vi "5_1.vi"() -> ()   [LabVIEW 2025, in "2023.lvlib"]
uses:
  2023.lvlib
  <vilib>/Utility/miscctls.llb/LVMapReplaceAction.ctl
  <userlib>/_OpenG.lib/string/string.llb/openg_string.lvlib
panel:
  out "Numeric 2":i32
  out "Map":T1(c390)
  out "64bit integer":i64[](array[numeric])
  out "Numeric":i32
  out "min value":i64
  out "subarray":i64[](array[numeric])
  out "Array 4":i64[][](array[numeric])
  out "Array":string[](array[string])
  out "lines":string[](array[string])
  in  "DEMO / REAL input":bool
  # "too low"
  # "485430760"
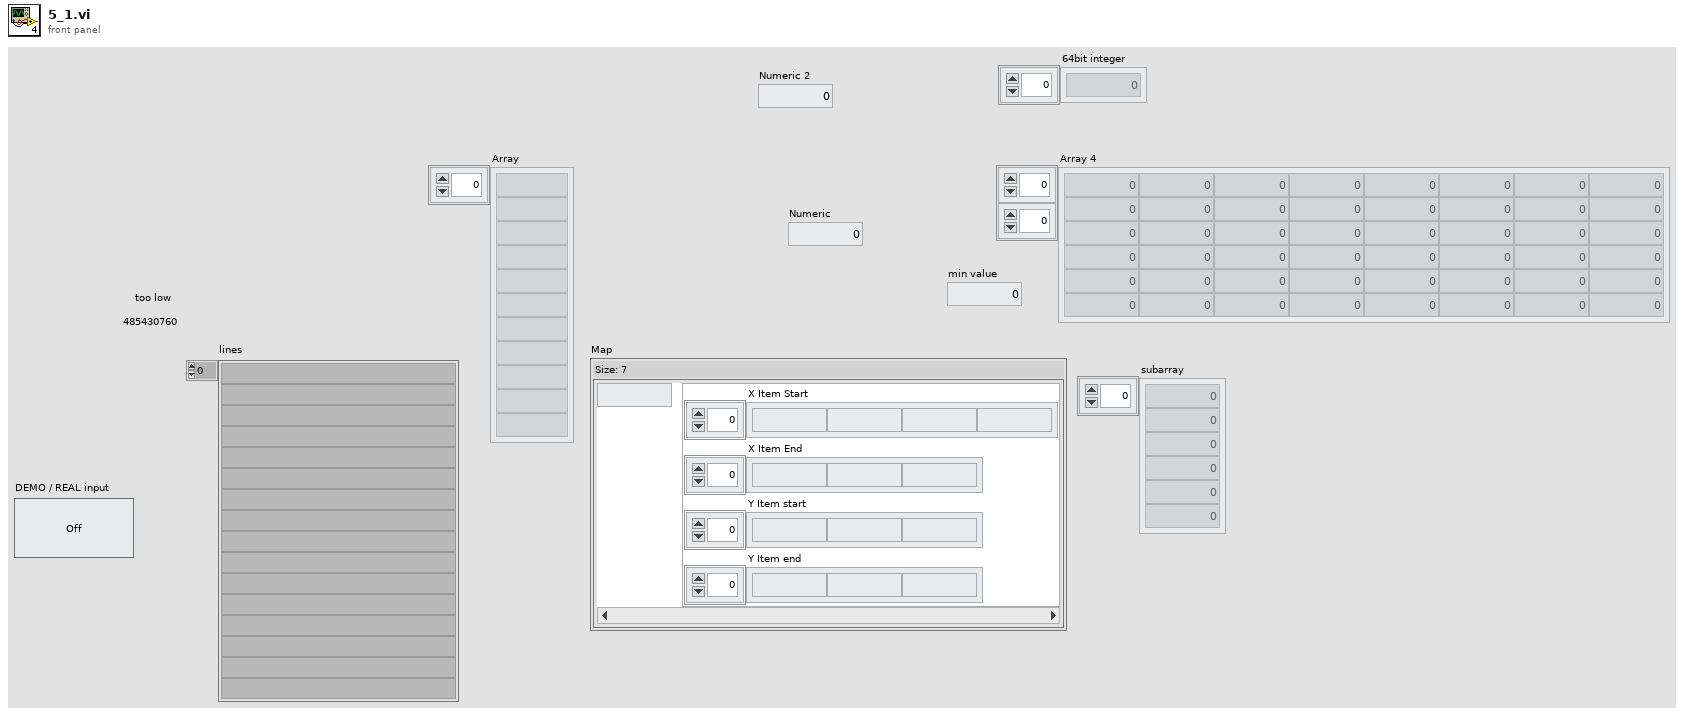
[diagram p1: front panel]
types:
  T1 = map{i32, cluster{"X Item Start":i64[], "X Item End":i64[], "Y Item start":i64[], "Y Item end":i64[]}}
  T2 = typedef "LVMapReplaceAction.ctl" = enum32{"Modify Entry only if found", "Add or Modify Entry", "Delete Entry"}
  T3 = cluster{"X Item Start":i64[], "X Item End":i64[], "Y Item start":i64[], "Y Item end":i64[]}
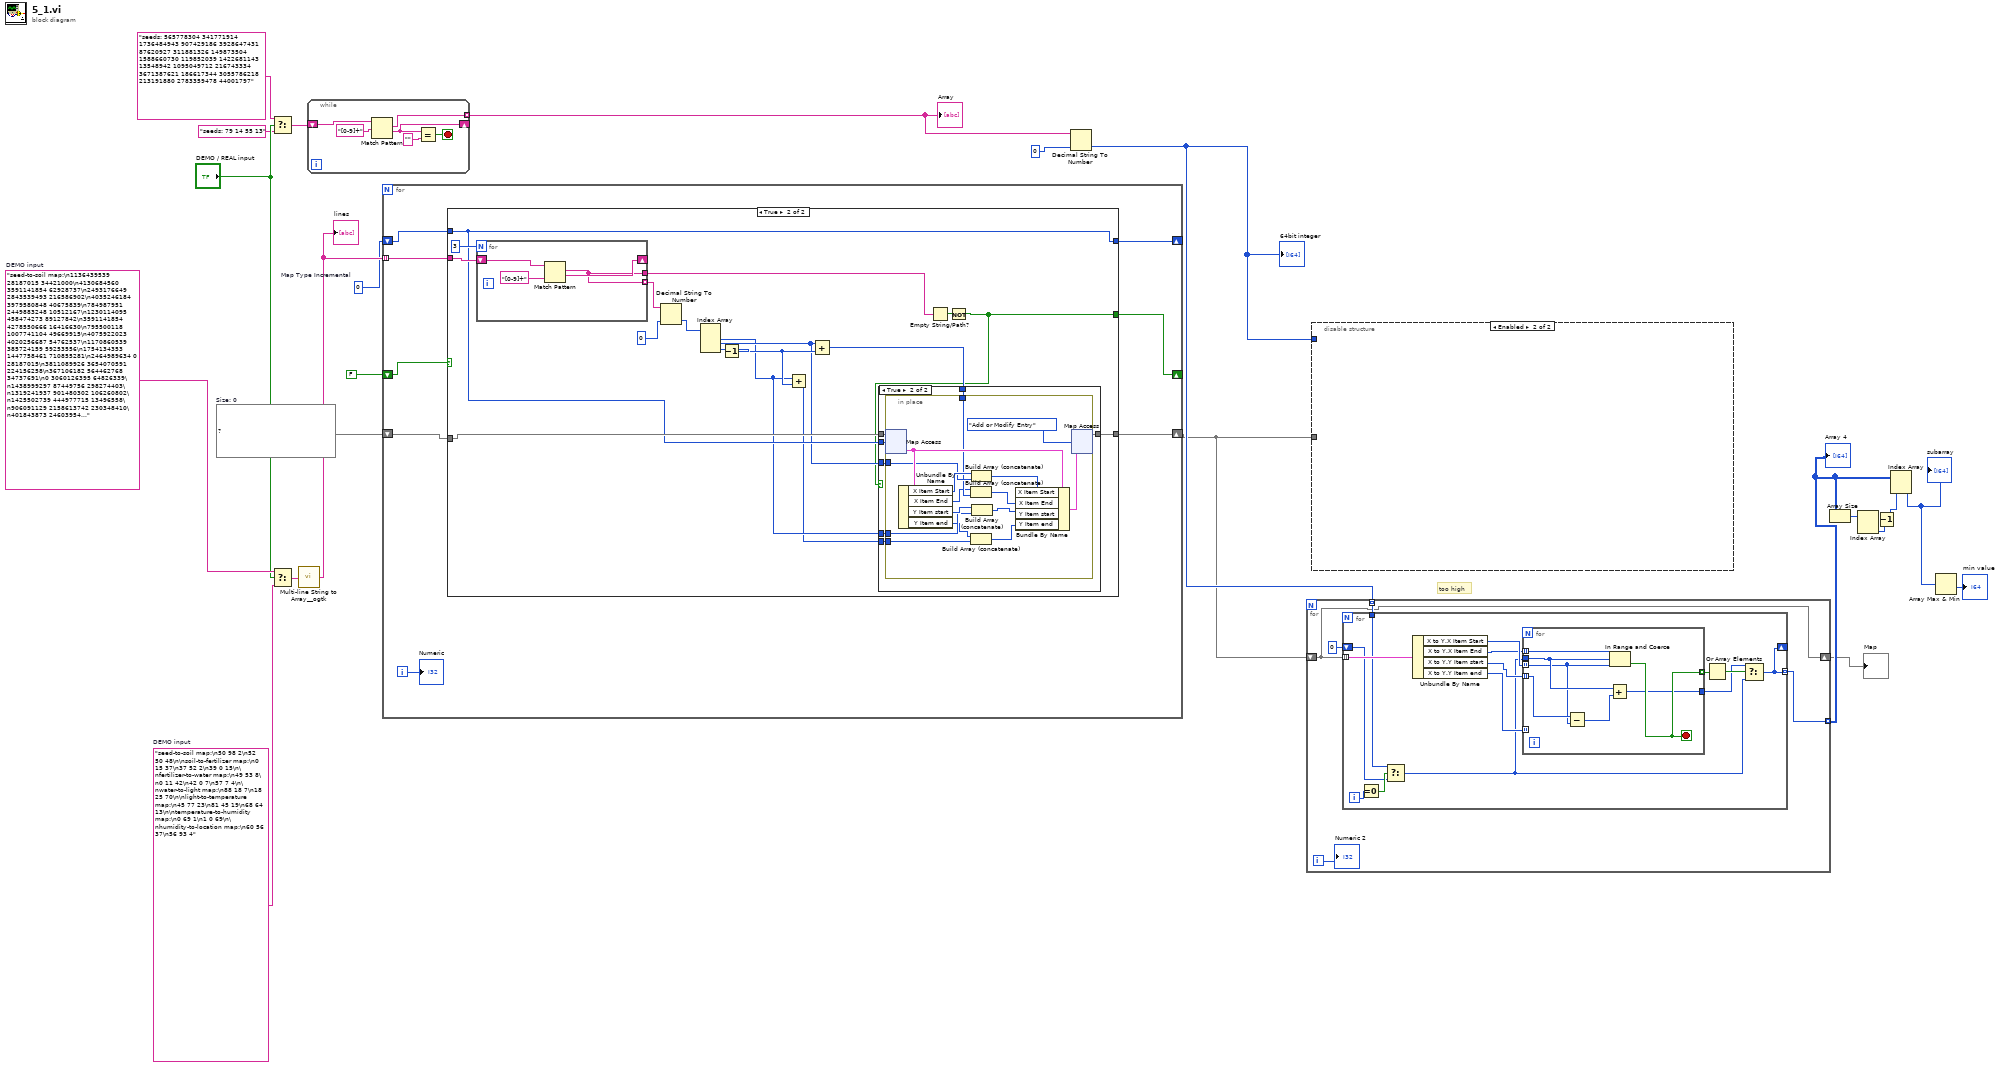
[diagram p0: block diagram]
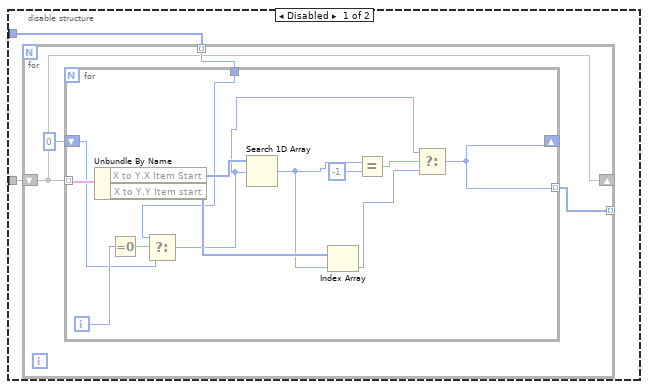
[diagram p2: hidden frame]
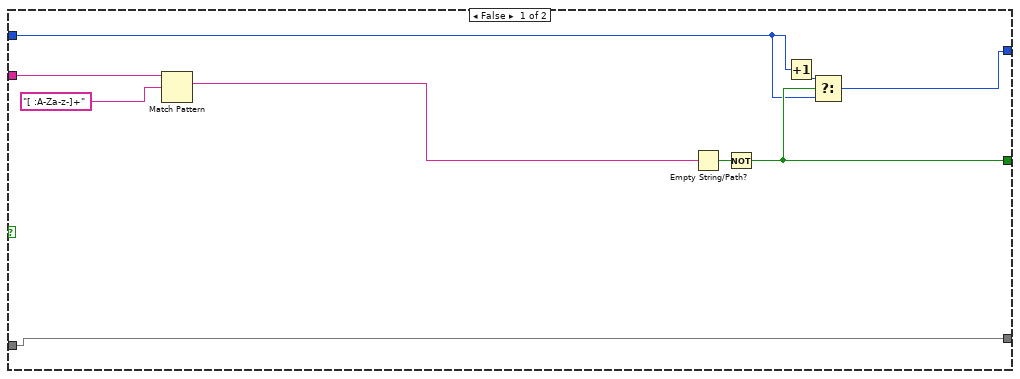
[diagram p3: hidden frame]
diagram:
  w11 = 0  # Map Type Incremental
  w13 = T1 {}  # Size: 0
  w22 = "seed-to-soil map:\n1136439539 28187015 34421000\n4130684560 3591141854 62928737\n2493176649 2843539493 216586902\n4035246184 3979580848 40675839\n784987951 2449883248 10512167\n1230114095 458474273 89127842\n3591141854 4278550666 16416630\n795500118 1007741104 49669915\n4075922023 4020256687 54762537\n1170860539 385724159 59253556\n1754134353 1447758461 710855281\n2464989634 0 28187015\n3811089926 3654070591 224156258\n367106182 564462768 34737691\n0 3060126395 64826339\n1438999297 87449756 298274403\n1319241937 901480302 106260802\n1425502739 444977715 13496558\n906091129 2158613742 230348410\n401843873 2460395415 383144078\n1737273700 547602115 16860653\n64826339 599200459 302279843\n2709763551 1057411019 390347442\n845170033 2388962152 60921096\n3607558484 4075019224 203531442\n3100110993 3124952734 265337006\n4193613297 3878226849 101353999\n3365447999 62608015 24841741\n\nsoil-to-fertilizer map:\n2997768542 2385088490 141138894\n2483957796 2361581050 23507440\n98641524 1346083581 385280737\n3138907436 2256873732 8670947\n0 2158232208 98641524\n3147578383 2265544679 96036371\n1035235183 2879344429 108036359\n2567031012 2526227384 63435416\n740156227 2589662800 180702628\n2630466428 1790930094 367302114\n1029837856 0 5397327\n1143271542 5397327 1340686254\n483922261 2987380788 256233966\n2507465236 1731364318 59565776\n920858855 2770365428 108979001\n\nfertilizer-to-water map:\n1539871014 1431400479 38399903\n4189242304 3947275099 105724992\n2012473116 0 61612686\n3673653298 3769966020 177309079\n25380533 833117788 21807501\n143369400 1411638591 19761888\n2698209531 61612686 40666379\n401367210 2888296065 27849039\n3850962377 4057978463 170640183\n1076364770 854925289 39443942\n0 2048878915 25380533\n2682826842 1483785677 15382689\n4026580932 4228618646 66348650\n790899137 2074259448 70405647\n2738875910 2609016218 230235412\n2090748148 1854132037 12185242\n163131288 1499168366 238235922\n1115808712 3002097202 63461270\n545943998 1215727887 195910704\n4092929582 3673653298 96312722\n1000530579 3065558472 75834191\n2074085802 2916145104 16662346\n429216249 1737404288 116727749\n1578270917 2174814019 434202199\n2969111322 102279065 44844471\n1179269982 669063687 164054101\n2463111278 507301424 161762263\n741854702 2839251630 49044435\n3013955793 894369231 236513741\n861304784 2144665095 30148924\n1525885719 1469800382 13985295\n132032949 2932807450 11336451\n2102933390 147123536 360177888\n47188034 1130882972 84844915\n4021602560 4053000091 4978372\n2624873541 2944143901 57953301\n891453708 3141392663 109076871\n1343324083 1866317279 182561636\n\nwater-to-light map:\n1509583382 1639808290 20361832\n3841220400 2799952377 116887408\n1472887638 3349716751 36695744\n1375316591 4197396249 97571047\n1030032900 38536653 44339012\n3776233310 1557050237 64987090\n1857053855 3386412495 71799907\n2963593546 2694182899 38493443\n3758462347 1622037327 17770963\n1018869652 82875665 11163248\n1308040556 2732676342 67276035\n1928853762 3953749938 243646311\n2488961036 3503789336 239267964\n3562290347 3458212402 6096433\n3568386780 1308040556 190075567\n2728229000 1997029610 235364546\n215668494 0 38536653\n1646361217 3743057300 109790942\n1529945214 3233300748 116416003\n1756152159 3852848242 100901696\n3958107808 1660170122 336859488\n3503356233 1498116123 58934114\n254205147 552157437 522214475\n3002086989 3464308835 39480501\n776419622 94038913 242450030\n2172500073 2916839785 316460963\n0 336488943 215668494\n3041567490 2232394156 461788743\n\nlight-to-temperature map:\n3498288578 2645051323 42074132\n608593503 673232568 65024140\n0 1287033796 108723708\n3979313387 3634135302 315653909\n2652759587 3018896130 103365881\n1093544955 942695289 7961217\n2756125468 3501628238 132507064\n419683046 1625547778 126722533\n683243352 349510049 26140330\n1101506172 511314709 142580382\n1283347805 375650379 135664330\n673617643 24016268 9625709\n709383682 1238532395 48501401\n3763762608 2402322728 184668443\n3948431051 2621479653 23571670\n3660408219 2687125455 102463666\n3561232935 2586991171 34488482\n2459767392 3122262011 192992195\n1244086554 1754618583 31645052\n1073753155 1497748002 19791800\n3972002721 3949789211 7310666\n3540362710 4077337854 20870225\n1419012135 738256708 79984976\n1746461061 1457945428 39802574\n3595721417 4190079809 64686802\n1616767336 653895091 19337477\n1275731606 823578131 7616199\n108723708 818241684 5336447\n546405579 1395757504 62187924\n1498997111 950656506 117770225\n2888632532 3957099877 102103275\n1744112789 1752270311 2348272\n2233819388 2077946837 225948004\n3762871885 2401432005 890723\n2136282224 2303894841 97537164\n3311914546 3315254206 186374032\n2118147522 4059203152 18134702\n308182087 831194330 111500959\n114060155 0 24016268\n2077946837 4254766611 40200685\n971525741 33641977 102227414\n1636104813 1517539802 108007976\n138076423 1068426731 170105664\n3220042816 4098208079 91871730\n2990735807 2789589121 229307009\n757885083 135869391 213640658\n\ntemperature-to-humidity map:\n1130946446 972737563 146373650\n1277320096 1760175559 41760032\n4151385320 4147641404 143581976\n2634337722 0 466605084\n1992884166 956487184 16250379\n4147641404 4291223380 3743916\n641064346 466605084 489882100\n1319080128 1801935591 673804038\n2009134545 2475739629 625203177\n0 1119111213 641064346\n\nhumidity-to-location map:\n3903940466 3635148971 125939893\n1458128760 2186815403 67353660\n3125319983 1458128760 728686643\n2261072201 3994982121 66012689\n3854006626 2992363154 49933840\n1525482420 3780550419 183145699\n2233668127 3967578047 27404074\n2442260515 3138011064 466023456\n740912129 0 327948845\n2422798960 3761088864 19461555\n1708628119 3963696118 3881929\n2327084890 3042296994 95714070\n4029880359 3604034520 31114451\n1712510048 2471205075 521158079\n367508399 695457244 373403730\n2908283971 2254169063 217036012\n0 327948845 367508399"  # DEMO input
  w21 = "seed-to-soil map:\n50 98 2\n52 50 48\n\nsoil-to-fertilizer map:\n0 15 37\n37 52 2\n39 0 15\n\nfertilizer-to-water map:\n49 53 8\n0 11 42\n42 0 7\n57 7 4\n\nwater-to-light map:\n88 18 7\n18 25 70\n\nlight-to-temperature map:\n45 77 23\n81 45 19\n68 64 13\n\ntemperature-to-humidity map:\n0 69 1\n1 0 69\n\nhumidity-to-location map:\n60 56 37\n56 93 4"  # DEMO input
  # "too high"
  n1 = Select(t="seeds: 565778304 341771914 1736484943 907429186 3928647431 87620927 311881326 149873504 1588660730 119852039 1422681143 13548942 1095049712 216743334 3671387621 186617344 3055786218 213191880 2783359478 44001797" ("element"), s="DEMO / REAL input", f="seeds: 79 14 55 13" ("element")) -> (s? t:f=w16:string)
  n2 = Select(t=w22, s="DEMO / REAL input", f=w21) -> (s? t:f=w20:string)
  n3 = call <userlib>:"Multi-line String to Array__ogtk.vi"("string"=w20) -> ("lines"=w15:string[])
  "lines" <- w15
  n4 = while {
    tunnel: [w26] -> w12 mode=indexing
    shift-right: [w23] -> _
    shift-left: w16 -> [w28]
    stop <- w24 stop-if-true
    n5 = Match Pattern(string=w28, regular expression="[0-9]+") -> (match substring=w26:string, after substring=w23:string)  [unwired: 1 in, 2 out]
    n6 = Equal?(x=w23, y="") -> (x = y?=w24:bool)
  }
  "Array" <- w12
  n7 = for {
    tunnel: w15 -> [w36] mode=indexing
    shift-right: [w35] -> _
    shift-left: FALSE -> [w34]
    shift-right: [w32] -> w4
    shift-left: w13 -> [w33]
    shift-right: [w31] -> _
    shift-left: w11 -> [w30]
    i -> [w29]
    n8 = case shown="True" w34 {
      tunnel: w36 -> [w44 w62]
      tunnel: [w40 w48] -> w35
      tunnel: w33 -> [w42 w58]
      tunnel: [w42 w56] -> w32
      tunnel: [w37 w55] -> w31
      tunnel: w30 -> [w38 w55]
      frame False {
        n9 = Match Pattern(string=w44, regular expression="[ :A-Za-z-]+") -> (match substring=w41:string)  [unwired: 1 in, 3 out]
        n10 = Empty String/Path?(string/path=w41) -> (empty?=w43:bool)
        n11 = Not(x=w43) -> (.not. x?=w40:bool)
        n12 = Increment(x=w38) -> (x+1=w39:i32)
        n13 = Select(t=w39, s=w40, f=w38) -> (s? t:f=w37:i32)
      }
      frame True {
        n14 = for {
          N: 3 -> [_]
          shift-right: [w87] -> _
          shift-left: w62 -> [w88]
          tunnel: [w86] -> w57
          tunnel: [w86] -> w59 mode=indexing
          n15 = Match Pattern(string=w88, regular expression="[0-9]+") -> (match substring=w86:string, after substring=w87:string)  [unwired: 1 in, 2 out]
        }
        n16 = Decimal String To Number(string=w59, default (0L)=i64 0 ("element")) -> (number=w46:i64[])  [unwired: 1 in, 1 out]
        n17 = Index Array(array=w46) -> (element #1=w51:i64, element #2=w52:i64, element #3=w54:i64)  [unwired: 3 in]
        n18 = Decrement(x=w54) -> (x-1=w53:i64)
        n19 = Add(x=w51, y=w53) -> (x+y=w49:i64)
        n20 = Add(x=w52, y=w53) -> (x+y=w50:i64)
        n21 = Empty String/Path?(string/path=w57) -> (empty?=w61:bool)
        n22 = Not(x=w61) -> (.not. x?=w48:bool)
        n23 = case shown="True" w48 {
          tunnel: w58 -> [w63 w70]
          tunnel: [w63 w69] -> w56
          tunnel: w55 -> [_ w68]
          tunnel: w52 -> [_ w67]
          tunnel: w51 -> [_ w66]
          tunnel: w50 -> [_ w65]
          tunnel: w49 -> [_ w64]
          frame False {
          }
          frame True {
            n24 = in-place {
              in-place-border: w67 -> [w78]
              in-place-border: w66 -> [w77]
              in-place-border: w65 -> [w76]
              in-place-border: w64 -> [w71]
              n25 = in-place-map #1(w70, w68) -> (w85:T3)  [unwired: 1 in, 1 out]
              n26 = Unbundle By Name(w85) -> ("X Item Start"=w84:i64[], "X Item End"=w75:i64[], "Y Item start"=w79:i64[], "Y Item end"=w73:i64[])
              n27 = Build Array (concatenate)(w75, w76) -> (w74:i64[])
              n28 = Build Array (concatenate)(w73, w71) -> (w72:i64[])
              n29 = Build Array (concatenate)(w84, w78) -> (w83:i64[])
              n30 = Build Array (concatenate)(w79, w77) -> (w80:i64[])
              n31 = Bundle By Name(cluster=w85, "X Item Start"=w83, "X Item End"=w74, "Y Item start"=w80, "Y Item end"=w72) -> (w82:T3)
              n32 = in-place-map #1(w82, LVMapReplaceAction."Add or Modify Entry" ("action")) -> (w69:T1)  [unwired: 2 out]
            }
          }
        }
      }
    }
    "Numeric" <- w29
  }
  n33 = Decimal String To Number(string=w12, default (0L)=i64 0 ("element")) -> (number=w5:i64[])  [unwired: 1 in, 1 out]
  "64bit integer" <- w5
  n34 = for {
    tunnel: w5 -> [w94] mode=indexing
    shift-right: [w91] -> w2
    shift-left: w4 -> [w91]
    tunnel: [w92] -> w3 mode=indexing
    i -> [w90]
    n35 = for {
      tunnel: w94 -> [w97]
      tunnel: w91 -> [w108] mode=indexing
      tunnel: [w101] -> w92 mode=indexing
      shift-right: [w101] -> _
      shift-left: i64 0 ("element") -> [w96]
      i -> [w99]
      n36 = Equal To 0?(x=w99) -> (x = 0?=w98:bool)
      n37 = Select(t=w97, s=w98, f=w96) -> (s? t:f=w95:i64)
      n38 = Unbundle By Name(w108) -> ("X to Y.X Item Start"=w107:i64[], "X to Y.X Item End"=w106:i64[], "X to Y.Y Item start"=w105:i64[], "X to Y.Y Item end"=w104:i64[])
      n39 = for {
        tunnel: w107 -> [w109] mode=indexing
        tunnel: w106 -> [w111] mode=indexing
        tunnel: w95 -> [w114]
        tunnel: w105 -> [w112] mode=indexing
        tunnel: w104 -> [_] mode=indexing
        tunnel: [w115] -> w103 mode=indexing
        tunnel: [w113] -> w100
        stop <- w115 stop-if-true
        n40 = Subtract(x=w112, y=w109) -> (x-y=w110:i64)
        n41 = Add(x=w114, y=w110) -> (x+y=w113:i64)
        n42 = In Range and Coerce(upper limit=w111, x=w114, lower limit=w109) -> (In Range?=w115:bool)  [unwired: 1 out]
      }
      n43 = Or Array Elements(Boolean array=w103) -> (logical OR=w102:bool)
      n44 = Select(t=w100, s=w102, f=w95) -> (s? t:f=w101:i64)
    }
    "Numeric 2" <- w90
  }
  "Array 4" <- w3
  "Map" <- w2
  n45 = disable-structure shown="Enabled" {
    disable-tunnel: w4 -> [w117 _]
    disable-tunnel: w5 -> [w116 _]
    frame Disabled {
      n46 = for {
        shift-right: [w120] -> _
        shift-left: w117 -> [w120]
        tunnel: w116 -> [w121] mode=indexing
        tunnel: [w119] -> _ mode=indexing
        n47 = for {
          tunnel: w120 -> [w134] mode=indexing
          tunnel: w121 -> [w124]
          tunnel: [w127] -> w119 mode=indexing
          shift-right: [w127] -> _
          shift-left: u32 0 ("element") -> [w123]
          i -> [w125]
          n48 = Unbundle By Name(w134) -> ("X to Y.X Item Start"=w133:i64[], "X to Y.Y Item start"=w132:i64[])
          n49 = Equal To 0?(x=w125) -> (x = 0?=w126:bool)
          n50 = Select(t=w124, s=w126, f=w123) -> (s? t:f=w122:i64)
          n51 = Search 1D Array(1D array=w133, element=w122) -> (index of element=w131:i32)  [unwired: 1 in]
          n52 = Index Array(array=w132, index=w131) -> (element=w128:i64)
          n53 = Equal?(x=w131, y=-1) -> (x = y?=w129:bool)
          n54 = Select(t=w122, s=w129, f=w128) -> (s? t:f=w127:i64)
        }
      }
    }
    frame Enabled {
    }
  }
  n55 = Array Size(array=w3) -> (size(s)=w10:i32[])
  n56 = Index Array(array=w10) -> (element #2=w9:i32)  [unwired: 2 in, 1 out]
  n57 = Decrement(x=w9) -> (x-1=w8:i32)
  n58 = Index Array(array=w3, index (col)=w8) -> (element=w7:i64[])  [unwired: 1 in]
  "subarray" <- w7
  n59 = Array Max & Min(array=w7) -> (min value=→"min value":i64)  [unwired: 3 out]
